vi "monitor_voltage.vi"() -> ()   [LabVIEW 2017]
uses:
  <vilib>/Instr/_visa.llb/VISA Configure Serial Port (Instr).vi
panel:
  in  "温度点维持时间（s）":dbl=30.0
  out "结束":bool
  in  "温度点（℃）":dbl[](array[numeric])=[70.0, 20.0, -40.0, -55.0, -40.0, 20.0, 70.0]
  in  "HP34401":refnum<visa-resource-name>
  out "XY图":cluster{dbl[], dbl[]}(graph)
  out "存储路径":string
  out "显示数据":i32(listbox)
  out "数据":string[][](array[string])
  in  "温度校验次数":dbl
  in  "实时温度(℃)":dbl
  in  "最低温度(℃)":dbl=-60.0
  in  "最高温度(℃)":dbl=75.0
  out "GWS":bool
  in  "GWS":refnum<visa-resource-name>
  in  "设定温度 (℃)":dbl
  in  "取点间隔 (S)":dbl
  in  "停止":bool
  in  "开始":bool
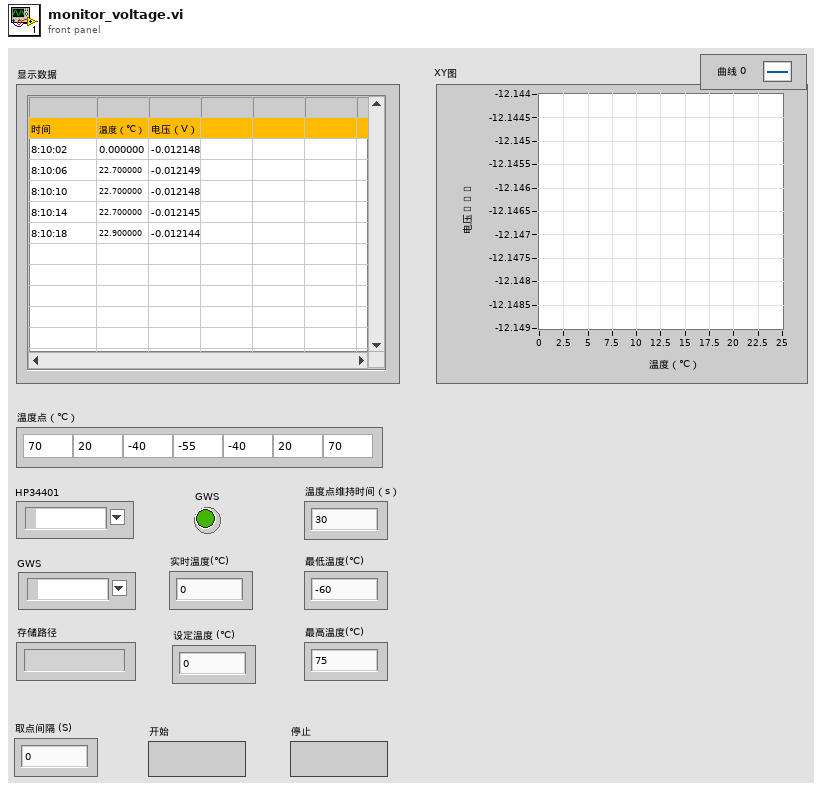
[diagram p1: front panel]
types:
  T1 = enum16{"open", "open or create", "create or replace", "create", "open (read-only)"}
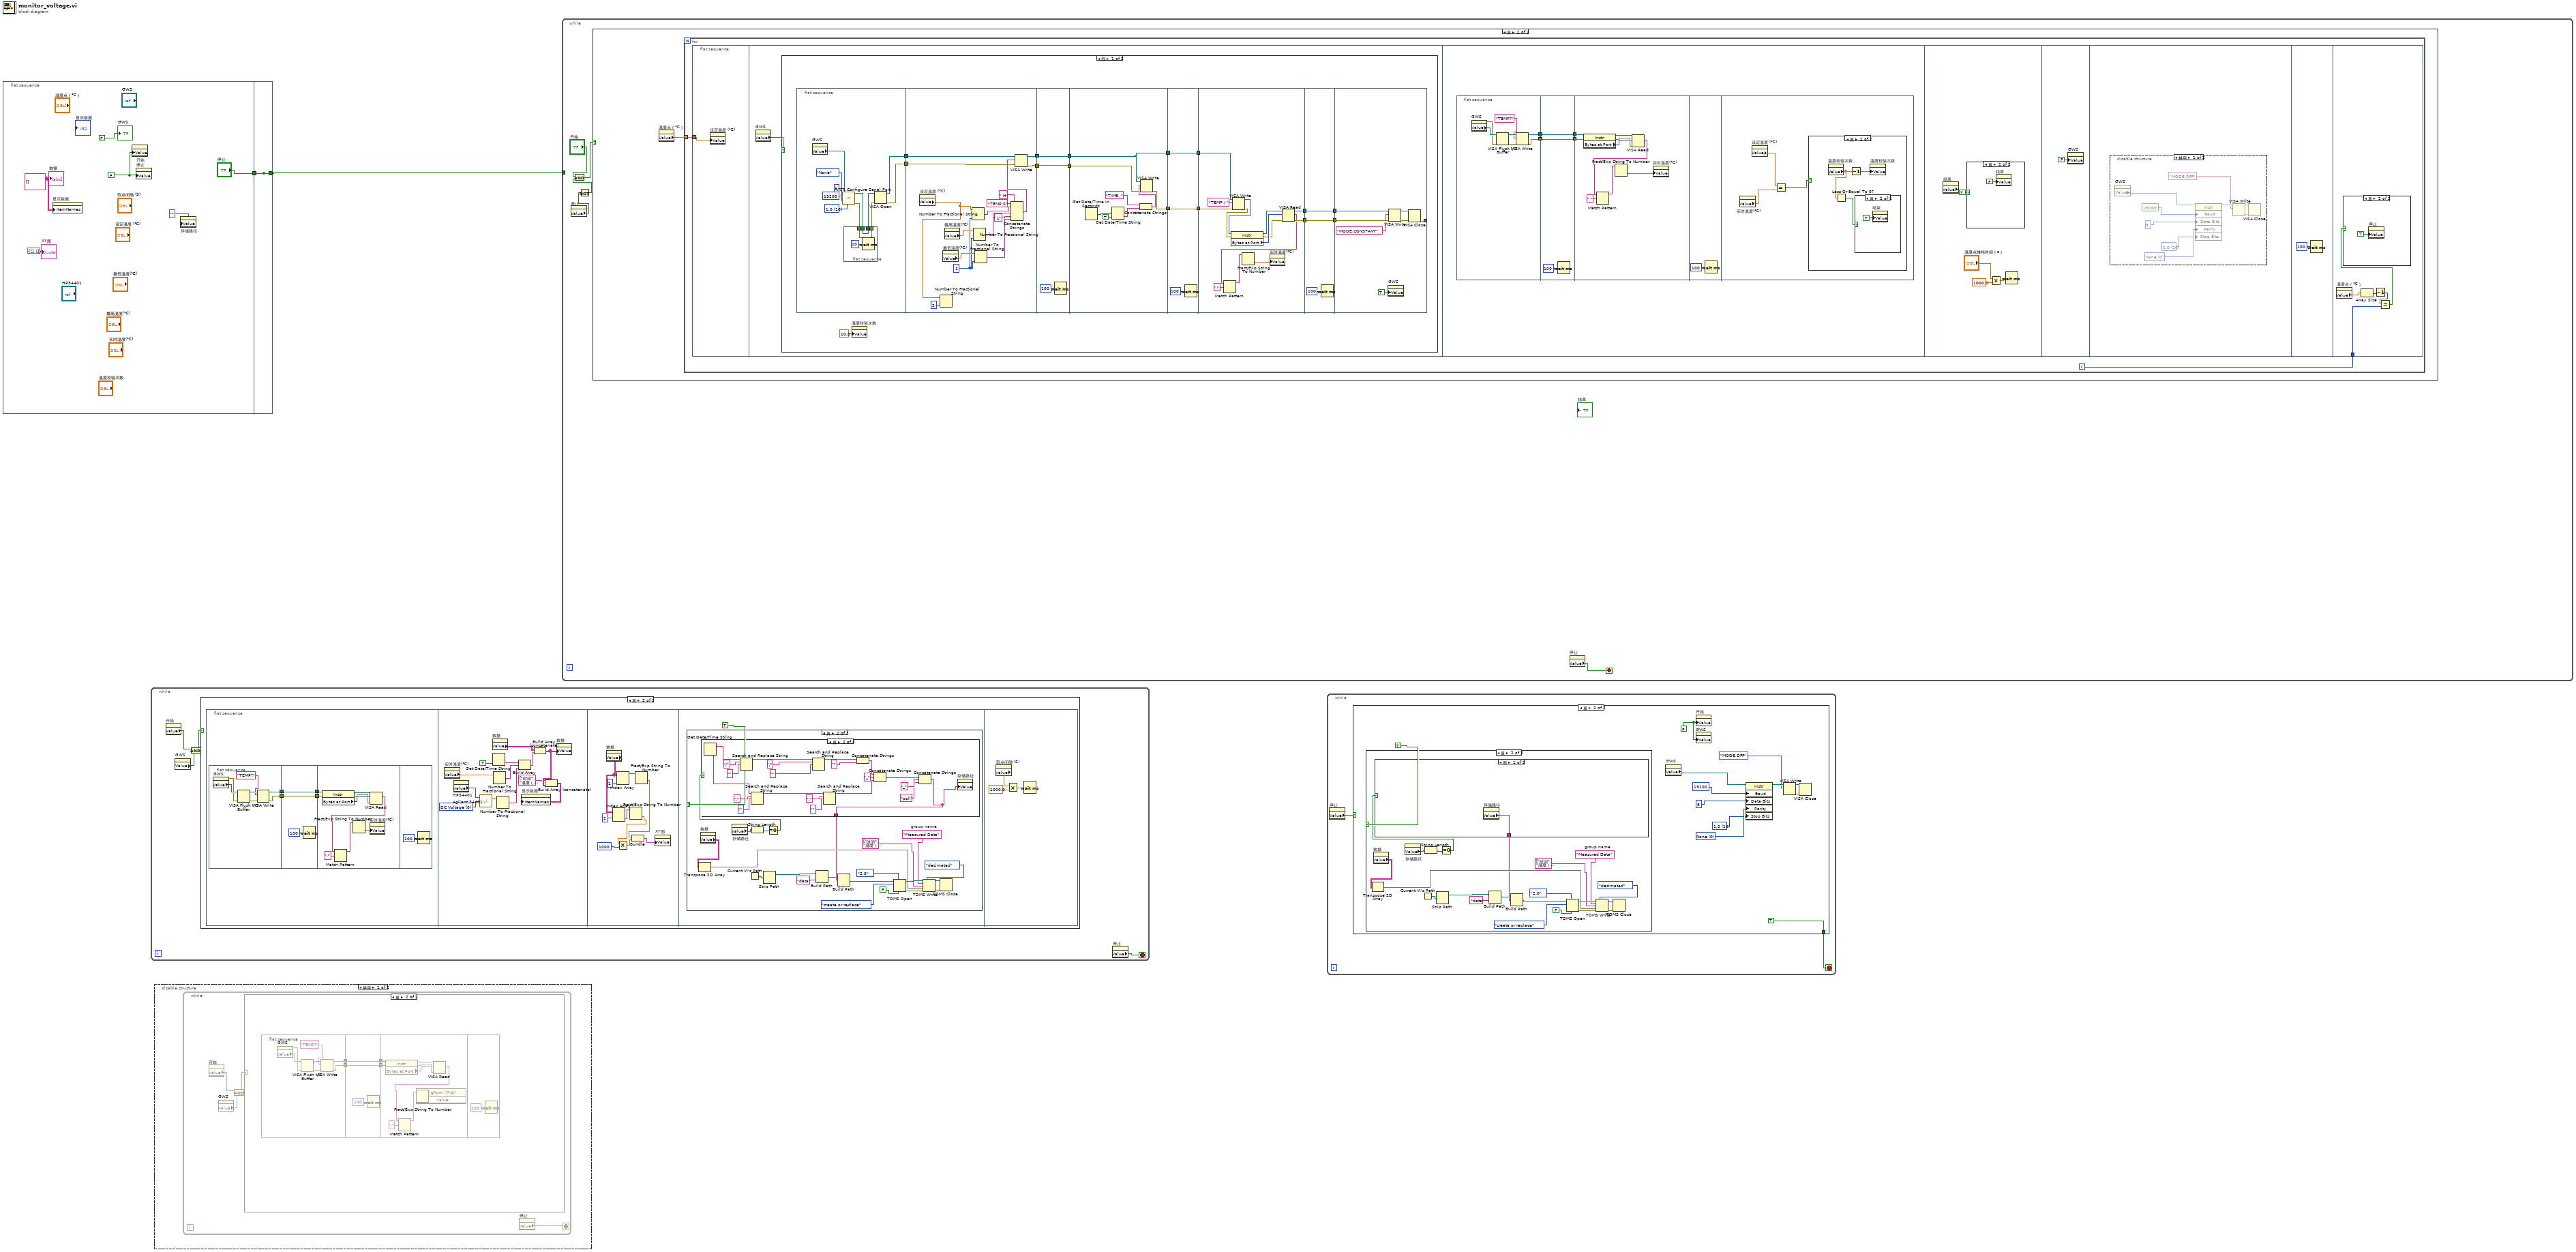
[diagram p0: block diagram]
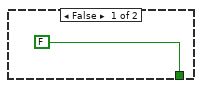
[diagram p4: hidden frame]
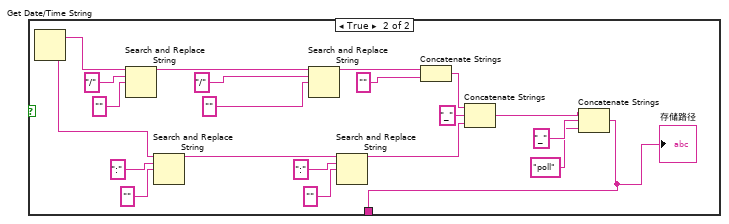
[diagram p6: hidden frame]
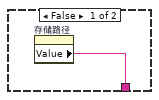
[diagram p9: hidden frame]
diagram:
  n1 = flat-sequence {
    tunnel: ["停止"] -> w2
    tunnel: [w9] -> _
    tunnel: w2 -> [w9]
    tunnel: [w9] -> w1
    frame #0 {
      w5 = FALSE ("停止")
      w8 = string[][] [] ("数据")
      n2 = property on="显示数据" class="MCListbox (严格)"("ItemNames"=w8) -> ()  [unwired: 2 in, 2 out]
      n3 = property on="开始" class="Bool (严格)"("Value"=w5) -> ()  [unwired: 2 in, 2 out]
      n4 = property on="停止" class="Bool (严格)"("Value"=w5) -> ()  [unwired: 2 in, 2 out]
      n5 = property on="存储路径" class="Str"("Value"="" ("存储路径")) -> ()  [unwired: 2 in, 2 out]
      "GWS" <- FALSE ("GWS")
      "数据" <- w8
      "XY图" <- cluster{dbl[], dbl[]} {[], []}
    }
    frame #1 {
    }
  }
  n6 = while {
    stop <- w10 stop-if-true
    n7 = property on="开始" class="Bool (严格)"() -> ("Value"=w11:bool)  [unwired: 2 in, 2 out]
    n8 = property on="GWS" class="Bool (严格)"() -> ("Value"=w13:bool)  [unwired: 2 in, 2 out]
    n9 = And(x=w11, y=w13) -> (x .and. y?=w12:bool)
    n10 = case shown="真" w12 {
      frame False {
      }
      frame True {
        n11 = flat-sequence {
          frame #0 {
            n12 = flat-sequence {
              tunnel: [w19] -> w17
              tunnel: [w18] -> w16
              tunnel: [w26] -> w15
              tunnel: w17 -> [w26]
              tunnel: [w25] -> w14
              tunnel: w16 -> [w25]
              tunnel: w15 -> [w36]
              tunnel: w14 -> [w35]
              frame #0 {
                n13 = property on="GWS" class="VISAName"() -> (error out=w23:errorcluster, "Value"=w24:refnum<visa-resource-name>)  [unwired: 2 in, 1 out]
                n14 = VISA Flush I/O Buffer(VISA resource name=w24, error in (no error)=w23) -> (VISA resource name out=w21:refnum<visa-resource-name>, error out=w22:errorcluster)  [unwired: 1 in]
                n15 = VISA Write(VISA resource name=w21, write buffer="TEMP?" ("写入缓冲区"), error in (no error)=w22) -> (VISA resource name out=w19:refnum<visa-resource-name>, error out=w18:errorcluster)  [unwired: 1 out]
              }
              frame #1 {
                n16 = Wait (ms)(milliseconds to wait=u32 100 ("等待时间（毫秒）")) -> ()  [unwired: 1 out]
              }
              frame #2 {
                n17 = property class="Instr"(reference=w36, error in=w35) -> (reference out=w34:refnum<visa-resource-name>, error out=w32:errorcluster, "Bytes at Port"=w33:u32)
                n18 = VISA Read(VISA resource name=w34, byte count=w33, error in (no error)=w32) -> (read buffer=w29:string)  [unwired: 3 out]
                n19 = Match Pattern(string=w29, regular expression="," ("正则表达式")) -> (before substring=w28:string)  [unwired: 1 in, 3 out]
                n20 = Fract/Exp String To Number(string=w28) -> (number=w31:dbl)  [unwired: 3 in, 1 out]
                n21 = property on="实时温度(℃)" class="DigNum (严格)"("Value"=w31) -> ()  [unwired: 2 in, 2 out]
              }
              frame #3 {
                n22 = Wait (ms)(milliseconds to wait=u32 100 ("等待时间（毫秒）")) -> ()  [unwired: 1 out]
              }
            }
          }
          frame #1 {
            w40 = u16 0 items=["DC Voltage", "AC Voltage", "2 - Wire Resistance", "4 - Wire Resistance", "DC Current", "AC Current", "Frequency", "Period", "Continuity", "Diode Checking", "VDC:VDC Ratio", "Temperature", "Capacitance"] ("Function (0: DC Voltage)")
            n23 = property on="实时温度(℃)" class="DigNum (严格)"() -> ("Value"=w49:dbl)  [unwired: 2 in, 2 out]
            n24 = property on="HP34401" class="VISAName"() -> ("Value"=w38:refnum<visa-resource-name>)  [unwired: 2 in, 2 out]
            n25 = call "Agilent 34401.vi"("Function (0: DC Voltage)"=w40, "VISA resource name"=w38) -> ("Measurement"=w50:dbl)  [unwired: 1 in, 1 out]
            n26 = property on="数据" class="Arr (严格)"() -> ("Value"=w44:string[][])  [unwired: 2 in, 2 out]
            n27 = Get Date/Time String(want seconds? (F)=TRUE ("disable buffering (T)")) -> (time string=w48:string)  [unwired: 2 in, 1 out]
            n28 = Number To Fractional String(number=w49) -> (F-format string=w47:string)  [unwired: 3 in]
            n29 = Number To Fractional String(number=w50) -> (F-format string=w46:string)  [unwired: 3 in]
            n30 = Build Array(w48, w47, w46) -> (w45:string[])
            n31 = Build Array (concatenate)(w44, w45) -> (w43:string[][])
            n32 = Build Array (concatenate)(string[] ["时间", "温度（℃）", "电压（V）"], w43) -> (w42:string[][])
            n33 = property on="显示数据" class="MCListbox (严格)"("ItemNames"=w42) -> ()  [unwired: 2 in, 2 out]
            n34 = property on="数据" class="Arr (严格)"("Value"=w43) -> ()  [unwired: 2 in, 2 out]
          }
          frame #2 {
            n35 = property on="数据" class="Arr (严格)"() -> ("Value"=w59:string[][])  [unwired: 2 in, 2 out]
            n36 = Index Array(array=w59, index (col)=2 ("禁用的索引 (列)")) -> (element=w55:string[])  [unwired: 1 in]
            n37 = Index Array(array=w59, index (col)=1 ("禁用的索引 (列)")) -> (element=w57:string[])  [unwired: 1 in]
            n38 = Fract/Exp String To Number(string=w55) -> (number=w52:dbl[])  [unwired: 3 in, 1 out]
            n39 = Multiply(x=w52, y=1000) -> (x*y=w53:dbl[])
            n40 = Fract/Exp String To Number(string=w57) -> (number=w56:dbl[])  [unwired: 3 in, 1 out]
            n41 = Bundle(w56, w53) -> (w54:cluster{dbl[], dbl[]})  [unwired: 1 in]
            n42 = property on="XY图" class="XYGraph (严格)"("Value"=w54) -> ()  [unwired: 2 in, 2 out]
          }
          frame #3 {
            n43 = case shown="真" TRUE {
              frame False {
              }
              frame True {
                w66 = "Measured Data"  # group name
                n44 = property on="数据" class="Arr (严格)"() -> ("Value"=w68:string[][])  [unwired: 2 in, 2 out]
                n45 = Transpose 2D Array(2D array=w68) -> (transposed array=w75:string[][])
                n46 = property on="存储路径" class="Str"() -> ("Value"=w65:string)  [unwired: 2 in, 2 out]
                n47 = Current VI's Path() -> (path=w69:path)
                n48 = String Length(string=w65) -> (length=w64:i32)
                n49 = Strip Path(path=w69) -> (stripped path=w79:path)  [unwired: 1 out]
                n50 = Equal To 0?(x=w64) -> (x = 0?=w63:bool)
                n51 = case shown="真" w63 {
                  tunnel: [w83 w84] -> w62
                  frame False {
                    n52 = property on="存储路径" class="Str"() -> ("Value"=w83:string)  [unwired: 2 in, 2 out]
                  }
                  frame True {
                    n53 = Get Date/Time String() -> (date string=w96:string, time string=w89:string)  [unwired: 3 in]
                    n54 = Search and Replace String(input string=w96, search string="/" ("搜索字符串"), replace string="" ("替换字符串(\"\")")) -> (result string=w102:string)  [unwired: 5 in, 3 out]
                    n55 = Search and Replace String(input string=w89, search string=":" ("搜索字符串"), replace string="" ("替换字符串(\"\")")) -> (result string=w93:string)  [unwired: 5 in, 3 out]
                    n56 = Search and Replace String(input string=w102, search string="/" ("搜索字符串"), replace string="" ("替换字符串(\"\")")) -> (result string=w99:string)  [unwired: 5 in, 3 out]
                    n57 = Search and Replace String(input string=w93, search string=":" ("搜索字符串"), replace string="" ("替换字符串(\"\")")) -> (result string=w88:string)  [unwired: 5 in, 3 out]
                    n58 = Concatenate Strings(w99, "" ("字符串")) -> (w97:string)
                    n59 = Concatenate Strings(w97, "_" ("字符串"), w88) -> (w86:string)
                    n60 = Concatenate Strings(w86, "_" ("字符串"), "poll" ("字符串")) -> (w84:string)
                    n61 = property on="存储路径" class="Str"("Value"=w84) -> ()  [unwired: 2 in, 2 out]
                  }
                }
                n62 = Build Path(base path=w79, name or relative path="data" ("字符串")) -> (appended path=w78:path)
                n63 = Build Path(base path=w78, name or relative path=w62) -> (appended path=w82:path)
                n64 = TDMS Open(6:FALSE ("disable buffering (T)"), 7:enum16{"1.0", "2.0"}."2.0" ("file format version (2.0)"), 10:T1."create or replace" ("operation"), 11:w82) -> (0:w80:errorcluster, 3:w77:refnum<k34>)  [unwired: 3 in]
                n65 = TDMS Write(0:w77, 1:enum16{"decimated", "interleaved"}."decimated" ("数据布局（0:降采样）"), 5:w66, 7:string[] ["时间", "温度（℃）", "电压（V）"], 9:w75, 11:w80) -> (4:w76:refnum<k34>, 15:w81:errorcluster)  [unwired: 2 out]
                n66 = TDMS Close(8:w81, 11:w76) -> ()  [unwired: 2 out]
              }
            }
          }
          frame #4 {
            n67 = property on="取点间隔 (S)" class="DigNum (严格)"() -> ("Value"=w107:dbl)  [unwired: 2 in, 2 out]
            n68 = Multiply(x=w107, y=1000.0) -> (x*y=w105:dbl)
            n69 = Wait (ms)(milliseconds to wait=w105) -> ()  [unwired: 1 out]
          }
        }
      }
    }
    n70 = property on="停止" class="Bool (严格)"() -> ("Value"=w10:bool)  [unwired: 2 in, 2 out]
  }
  n71 = disable-structure shown="禁用" {
    frame Disabled {
      n72 = while {
        stop <- w108 stop-if-true
        n73 = property on="开始" class="Bool (严格)"() -> ("Value"=w109:bool)  [unwired: 2 in, 2 out]
        n74 = property on="GWS" class="Bool (严格)"() -> ("Value"=w111:bool)  [unwired: 2 in, 2 out]
        n75 = And(x=w109, y=w111) -> (x .and. y?=w110:bool)
        n76 = case shown="真" w110 {
          frame False {
          }
          frame True {
            n77 = flat-sequence {
              tunnel: [w117] -> w115
              tunnel: [w116] -> w114
              tunnel: [w124] -> w113
              tunnel: w115 -> [w124]
              tunnel: [w123] -> w112
              tunnel: w114 -> [w123]
              tunnel: w113 -> [w134]
              tunnel: w112 -> [w133]
              frame #0 {
                n78 = property on="GWS" class="VISAName"() -> (error out=w121:errorcluster, "Value"=w122:refnum<visa-resource-name>)  [unwired: 2 in, 1 out]
                n79 = VISA Flush I/O Buffer(VISA resource name=w122, error in (no error)=w121) -> (VISA resource name out=w119:refnum<visa-resource-name>, error out=w120:errorcluster)  [unwired: 1 in]
                n80 = VISA Write(VISA resource name=w119, write buffer="TEMP?" ("写入缓冲区"), error in (no error)=w120) -> (VISA resource name out=w117:refnum<visa-resource-name>, error out=w116:errorcluster)  [unwired: 1 out]
              }
              frame #1 {
                n81 = Wait (ms)(milliseconds to wait=u32 100 ("等待时间（毫秒）")) -> ()  [unwired: 1 out]
              }
              frame #2 {
                n82 = property class="Instr"(reference=w134, error in=w133) -> (reference out=w132:refnum<visa-resource-name>, error out=w130:errorcluster, "Bytes at Port"=w131:u32)
                n83 = VISA Read(VISA resource name=w132, byte count=w131, error in (no error)=w130) -> (read buffer=w127:string)  [unwired: 3 out]
                n84 = Match Pattern(string=w127, regular expression="," ("正则表达式")) -> (before substring=w126:string)  [unwired: 1 in, 3 out]
                n85 = Fract/Exp String To Number(string=w126) -> (number=w129:dbl)  [unwired: 3 in, 1 out]
                n86 = property on="属性节点" class="DigNum (严格)"("Value"=w129) -> ()  [unwired: 2 in, 2 out]
              }
              frame #3 {
                n87 = Wait (ms)(milliseconds to wait=u32 100 ("等待时间（毫秒）")) -> ()  [unwired: 1 out]
              }
            }
          }
        }
        n88 = property on="停止" class="Bool (严格)"() -> ("Value"=w108:bool)  [unwired: 2 in, 2 out]
      }
    }
    frame Enabled {
    }
  }
  n89 = while {
    tunnel: w1 -> [_]
    stop <- w136 stop-if-true
    n90 = property on="停止" class="Bool (严格)"() -> ("Value"=w138:bool)  [unwired: 2 in, 2 out]
    n91 = Not(x=w138) -> (.not. x?=w137:bool)
    n92 = And(x="开始", y=w137) -> (x .and. y?=w139:bool)
    n93 = case shown="真" w139 {
      frame False {
      }
      frame True {
        n94 = property on="温度点（℃）" class="Arr (严格)"() -> ("Value"=w141:dbl[])  [unwired: 2 in, 2 out]
        n95 = for {
          tunnel: w141 -> [w142] mode=indexing
          i -> [w143]
          n96 = flat-sequence {
            tunnel: w142 -> [w144]
            tunnel: w143 -> [w277]
            frame #0 {
              n97 = property on="设定温度 (℃)" class="DigNum (严格)"("Value"=w144) -> ()  [unwired: 2 in, 2 out]
            }
            frame #1 {
              n98 = property on="GWS" class="Bool (严格)"() -> ("Value"=w145:bool)  [unwired: 2 in, 2 out]
              n99 = case shown="假" w145 {
                frame False {
                  n100 = flat-sequence {
                    tunnel: [w164] -> w160
                    tunnel: [w163] -> w159
                    tunnel: [w181] -> w158
                    tunnel: [w180] -> w157
                    tunnel: w160 -> [w178]
                    tunnel: w159 -> [w177]
                    tunnel: [w193] -> w156
                    tunnel: w158 -> [w193]
                    tunnel: [w192] -> w155
                    tunnel: w157 -> [w192]
                    tunnel: w156 -> [w195]
                    tunnel: w155 -> [w196]
                    tunnel: [w195] -> w154
                    tunnel: [w194] -> w153
                    tunnel: w154 -> [w203]
                    tunnel: [w203] -> w152
                    tunnel: [w202] -> w151
                    tunnel: w153 -> [w202]
                    tunnel: w152 -> [w216]
                    tunnel: w151 -> [w215]
                    tunnel: [w211] -> w150
                    tunnel: [w210] -> w149
                    tunnel: [w220] -> w148
                    tunnel: w150 -> [w220]
                    tunnel: w149 -> [w219]
                    tunnel: [w219] -> w147
                    tunnel: w148 -> [w227]
                    tunnel: w147 -> [w226]
                    tunnel: [w222] -> _
                    frame #0 {
                      w168 = u16 10 items=["1.0"=10, "1.5"=15, "2.0"=20] ("stop bits (10: 1 bit)")
                      n101 = property on="GWS" class="VISAName"() -> ("Value"=w167:refnum<visa-resource-name>)  [unwired: 2 in, 2 out]
                      n102 = call-poly "VISA Configure Serial Port"("VISA resource name"=w167, "baud rate (9600)"=u32 19200, "data bits (8)"=u16 8, "parity (0:none)"=enum16{"None", "Odd", "Even", "Mark", "Space"}."None", "stop bits (10: 1 bit)"=w168) -> ("VISA resource name out"=w162:refnum<visa-resource-name>, "error out"=w166:errorcluster)  [unwired: 9 in]
                      n103 = flat-sequence {
                        tunnel: w166 -> [w173]
                        tunnel: [w173] -> w165
                        tunnel: w162 -> [w172]
                        tunnel: [w172] -> w161
                        frame #0 {
                          n104 = Wait (ms)(milliseconds to wait=u32 20 ("等待时间（毫秒）")) -> ()  [unwired: 1 out]
                        }
                      }
                      n105 = VISA Open(error in (no error)=w165, VISA resource name=w161) -> (VISA resource name=w164:refnum<visa-resource-name>, error out=w163:errorcluster)  [unwired: 3 in]
                    }
                    frame #1 {
                      w185 = i16 1 ("精度(6)")
                      n106 = property on="设定温度 (℃)" class="DigNum (严格)"() -> ("Value"=w175:dbl)  [unwired: 2 in, 2 out]
                      n107 = Number To Fractional String(number=w175, precision (6)=i16 2 ("精度(6)")) -> ()  [unwired: 2 in, 1 out]
                      n108 = property on="最低温度(℃)" class="DigNum (严格)"() -> ("Value"=w187:dbl)  [unwired: 2 in, 2 out]
                      n109 = property on="最高温度(℃)" class="DigNum (严格)"() -> ("Value"=w186:dbl)  [unwired: 2 in, 2 out]
                      n110 = Number To Fractional String(number=w175, precision (6)=w185) -> (F-format string=w190:string)  [unwired: 2 in]
                      n111 = Number To Fractional String(number=w186, precision (6)=w185) -> (F-format string=w188:string)  [unwired: 2 in]
                      n112 = Number To Fractional String(number=w187, precision (6)=w185) -> (F-format string=w189:string)  [unwired: 2 in]
                      n113 = Concatenate Strings("TEMP,S" ("字符串"), w190, " H" ("字符串"), w188, " L" ("字符串"), w189) -> (w179:string)
                      n114 = VISA Write(VISA resource name=w178, write buffer=w179, error in (no error)=w177) -> (VISA resource name out=w181:refnum<visa-resource-name>, error out=w180:errorcluster)  [unwired: 1 out]
                    }
                    frame #2 {
                      n115 = Wait (ms)(milliseconds to wait=u32 100 ("等待时间（毫秒）")) -> ()  [unwired: 1 out]
                    }
                    frame #3 {
                      n116 = Get Date/Time In Seconds() -> (seconds since 1Jan1904=w199:timestamp)
                      n117 = Get Date/Time String(seconds (now)=w199, want seconds? (F)=TRUE ("需要秒？(F)")) -> (time string=w201:string)  [unwired: 1 in, 1 out]
                      n118 = Concatenate Strings("TIME, " ("字符串"), w201) -> (w197:string)
                      n119 = VISA Write(VISA resource name=w195, write buffer=w197, error in (no error)=w196) -> (error out=w194:errorcluster)  [unwired: 2 out]
                    }
                    frame #4 {
                      n120 = Wait (ms)(milliseconds to wait=u32 100 ("等待时间（毫秒）")) -> ()  [unwired: 1 out]
                    }
                    frame #5 {
                      n121 = VISA Write(VISA resource name=w216, write buffer="TEMP？" ("写入缓冲区"), error in (no error)=w215) -> (VISA resource name out=w217:refnum<visa-resource-name>, error out=w212:errorcluster)  [unwired: 1 out]
                      n122 = property class="Instr"(reference=w217, error in=w212) -> (reference out=w214:refnum<visa-resource-name>, error out=w209:errorcluster, "Bytes at Port"=w213:u32)
                      n123 = VISA Read(VISA resource name=w214, byte count=w213, error in (no error)=w209) -> (VISA resource name out=w211:refnum<visa-resource-name>, read buffer=w205:string, error out=w210:errorcluster)  [unwired: 1 out]
                      n124 = Match Pattern(string=w205, regular expression="," ("正则表达式")) -> (before substring=w206:string)  [unwired: 1 in, 3 out]
                      n125 = Fract/Exp String To Number(string=w206) -> (number=w208:dbl)  [unwired: 3 in, 1 out]
                      n126 = property on="实时温度(℃)" class="DigNum (严格)"("Value"=w208) -> ()  [unwired: 2 in, 2 out]
                    }
                    frame #6 {
                      n127 = Wait (ms)(milliseconds to wait=u32 100 ("等待时间（毫秒）")) -> ()  [unwired: 1 out]
                    }
                    frame #7 {
                      n128 = property on="GWS" class="Bool (严格)"("Value"=TRUE ("GWS")) -> ()  [unwired: 2 in, 2 out]
                      n129 = VISA Write(VISA resource name=w227, write buffer="MODE,CONSTANT" ("写入缓冲区"), error in (no error)=w226) -> (VISA resource name out=w224:refnum<visa-resource-name>, error out=w223:errorcluster)  [unwired: 1 out]
                      n130 = VISA Close(VISA resource name=w224, error in (no error)=w223) -> (error out=w222:errorcluster)
                    }
                  }
                  n131 = property on="温度校验次数" class="DigNum (严格)"("Value"=10.0 ("温度校验次数")) -> ()  [unwired: 2 in, 2 out]
                }
                frame True {
                }
              }
            }
            frame #2 {
              n132 = flat-sequence {
                tunnel: [w234] -> w232
                tunnel: [w233] -> w231
                tunnel: [w241] -> w230
                tunnel: w232 -> [w241]
                tunnel: [w240] -> w229
                tunnel: w231 -> [w240]
                tunnel: w230 -> [w251]
                tunnel: w229 -> [w250]
                frame #0 {
                  n133 = property on="GWS" class="VISAName"() -> (error out=w238:errorcluster, "Value"=w239:refnum<visa-resource-name>)  [unwired: 2 in, 1 out]
                  n134 = VISA Flush I/O Buffer(VISA resource name=w239, error in (no error)=w238) -> (VISA resource name out=w236:refnum<visa-resource-name>, error out=w237:errorcluster)  [unwired: 1 in]
                  n135 = VISA Write(VISA resource name=w236, write buffer="TEMP?" ("写入缓冲区"), error in (no error)=w237) -> (VISA resource name out=w234:refnum<visa-resource-name>, error out=w233:errorcluster)  [unwired: 1 out]
                }
                frame #1 {
                  n136 = Wait (ms)(milliseconds to wait=u32 100 ("等待时间（毫秒）")) -> ()  [unwired: 1 out]
                }
                frame #2 {
                  n137 = property class="Instr"(reference=w251, error in=w250) -> (reference out=w249:refnum<visa-resource-name>, error out=w247:errorcluster, "Bytes at Port"=w248:u32)
                  n138 = VISA Read(VISA resource name=w249, byte count=w248, error in (no error)=w247) -> (read buffer=w244:string)  [unwired: 3 out]
                  n139 = Match Pattern(string=w244, regular expression="," ("正则表达式")) -> (before substring=w243:string)  [unwired: 1 in, 3 out]
                  n140 = Fract/Exp String To Number(string=w243) -> (number=w246:dbl)  [unwired: 3 in, 1 out]
                  n141 = property on="实时温度(℃)" class="DigNum (严格)"("Value"=w246) -> ()  [unwired: 2 in, 2 out]
                }
                frame #3 {
                  n142 = Wait (ms)(milliseconds to wait=u32 100 ("等待时间（毫秒）")) -> ()  [unwired: 1 out]
                }
                frame #4 {
                  n143 = property on="实时温度(℃)" class="DigNum (严格)"() -> ("Value"=w255:dbl)  [unwired: 2 in, 2 out]
                  n144 = property on="设定温度 (℃)" class="DigNum (严格)"() -> ("Value"=w254:dbl)  [unwired: 2 in, 2 out]
                  n145 = Equal?(x=w254, y=w255) -> (x = y?=w253:bool)
                  n146 = case shown="真" w253 {
                    frame False {
                    }
                    frame True {
                      n147 = property on="温度校验次数" class="DigNum (严格)"() -> ("Value"=w256:dbl)  [unwired: 2 in, 2 out]
                      n148 = Less Or Equal To 0?(x=w256) -> (x <= 0?=w257:bool)
                      n149 = Decrement(x=w256) -> (x-1=w258:dbl)
                      n150 = case shown="真" w257 {
                        frame False {
                        }
                        frame True {
                          n151 = property on="结束" class="Bool (严格)"("Value"=TRUE ("结束")) -> ()  [unwired: 2 in, 2 out]
                        }
                      }
                      n152 = property on="温度校验次数" class="DigNum (严格)"("Value"=w258) -> ()  [unwired: 2 in, 2 out]
                    }
                  }
                }
              }
            }
            frame #3 {
              n153 = property on="结束" class="Bool (严格)" props=["Value"]() -> ()  [unwired: 2 in, 3 out]
              n154 = case shown="真" TRUE {
                frame False {
                }
                frame True {
                  n155 = property on="结束" class="Bool (严格)"("Value"=FALSE ("结束")) -> ()  [unwired: 2 in, 2 out]
                }
              }
              n156 = Multiply(x="温度点维持时间（s）", y=1000.0) -> (x*y=w261:dbl)
              n157 = Wait (ms)(milliseconds to wait=w261) -> ()  [unwired: 1 out]
            }
            frame #4 {
              n158 = property on="GWS" class="Bool (严格)"("Value"=FALSE ("结束")) -> ()  [unwired: 2 in, 2 out]
            }
            frame #5 {
              n159 = disable-structure shown="禁用" {
                frame Disabled {
                  w266 = u16 10 items=["1.0"=10, "1.5"=15, "2.0"=20] ("Serial Settings:Stop Bits")
                  w267 = u16 0 items=["None", "Odd", "Even", "Mark", "Space"] ("Serial Settings:Parity")
                  n160 = property on="GWS" class="VISAName"() -> ("Value"=w274:refnum<visa-resource-name>)  [unwired: 2 in, 2 out]
                  n161 = property class="Instr"(reference=w274, "Baud"=u32 19200 ("Serial Settings:Baud Rate"), "Data Bits"=u16 8 ("Serial Settings:Data Bits"), "Parity"=w267, "Stop Bits"=w266) -> (reference out=w271:refnum<visa-resource-name>)  [unwired: 1 in, 1 out]
                  n162 = VISA Write(VISA resource name=w271, write buffer="MODE,OFF" ("写入缓冲区")) -> (VISA resource name out=w273:refnum<visa-resource-name>, error out=w272:errorcluster)  [unwired: 1 in, 1 out]
                  n163 = VISA Close(VISA resource name=w273, error in (no error)=w272) -> ()  [unwired: 1 out]
                }
                frame Enabled {
                }
              }
            }
            frame #6 {
              n164 = Wait (ms)(milliseconds to wait=u32 100 ("等待时间（毫秒）")) -> ()  [unwired: 1 out]
            }
            frame #7 {
              n165 = property on="温度点（℃）" class="Arr (严格)"() -> ("Value"=w280:dbl[])  [unwired: 2 in, 2 out]
              n166 = Array Size(array=w280) -> (size(s)=w279:i32)
              n167 = Decrement(x=w279) -> (x-1=w278:i32)
              n168 = Equal?(x=w278, y=w277) -> (x = y?=w276:bool)
              n169 = case shown="真" w276 {
                frame False {
                }
                frame True {
                  n170 = property on="停止" class="Bool (严格)"("Value"=TRUE ("恒温开始")) -> ()  [unwired: 2 in, 2 out]
                }
              }
            }
          }
        }
      }
    }
    n171 = property on="停止" class="Bool (严格)"() -> ("Value"=w136:bool)  [unwired: 2 in, 2 out]
  }
  n172 = while {
    stop <- w282 stop-if-true
    n173 = property on="停止" class="Bool (严格)"() -> ("Value"=w283:bool)  [unwired: 2 in, 2 out]
    n174 = case shown="真" w283 {
      tunnel: [FALSE TRUE] -> w282
      frame False {
      }
      frame True {
        w287 = FALSE ("开始")
        w288 = u16 10 items=["1.0"=10, "1.5"=15, "2.0"=20] ("Serial Settings:Stop Bits")
        w289 = u16 0 items=["None", "Odd", "Even", "Mark", "Space"] ("Serial Settings:Parity")
        n175 = case shown="真" TRUE {
          frame False {
          }
          frame True {
            w301 = "Measured Data"  # group name
            n176 = property on="数据" class="Arr (严格)"() -> ("Value"=w303:string[][])  [unwired: 2 in, 2 out]
            n177 = Transpose 2D Array(2D array=w303) -> (transposed array=w310:string[][])
            n178 = property on="存储路径" class="Str"() -> ("Value"=w300:string)  [unwired: 2 in, 2 out]
            n179 = Current VI's Path() -> (path=w304:path)
            n180 = String Length(string=w300) -> (length=w299:i32)
            n181 = Strip Path(path=w304) -> (stripped path=w314:path)  [unwired: 1 out]
            n182 = Equal To 0?(x=w299) -> (x = 0?=w298:bool)
            n183 = case shown="假" w298 {
              tunnel: [w318 w319] -> w297
              frame False {
                n184 = property on="存储路径" class="Str"() -> ("Value"=w318:string)  [unwired: 2 in, 2 out]
              }
              frame True {
                n185 = Get Date/Time String() -> (date string=w331:string, time string=w324:string)  [unwired: 3 in]
                n186 = Search and Replace String(input string=w331, search string="/" ("搜索字符串"), replace string="" ("替换字符串(\"\")")) -> (result string=w337:string)  [unwired: 5 in, 3 out]
                n187 = Search and Replace String(input string=w324, search string=":" ("搜索字符串"), replace string="" ("替换字符串(\"\")")) -> (result string=w328:string)  [unwired: 5 in, 3 out]
                n188 = Search and Replace String(input string=w337, search string="/" ("搜索字符串"), replace string="" ("替换字符串(\"\")")) -> (result string=w334:string)  [unwired: 5 in, 3 out]
                n189 = Search and Replace String(input string=w328, search string=":" ("搜索字符串"), replace string="" ("替换字符串(\"\")")) -> (result string=w323:string)  [unwired: 5 in, 3 out]
                n190 = Concatenate Strings(w334, "" ("字符串")) -> (w332:string)
                n191 = Concatenate Strings(w332, "_" ("字符串"), w323) -> (w321:string)
                n192 = Concatenate Strings(w321, "_" ("字符串"), "poll" ("字符串")) -> (w319:string)
                "存储路径" <- w319
              }
            }
            n193 = Build Path(base path=w314, name or relative path="data" ("字符串")) -> (appended path=w313:path)
            n194 = Build Path(base path=w313, name or relative path=w297) -> (appended path=w317:path)
            n195 = TDMS Open(6:FALSE ("disable buffering (T)"), 7:enum16{"1.0", "2.0"}."2.0" ("file format version (2.0)"), 10:T1."create or replace" ("operation"), 11:w317) -> (0:w315:errorcluster, 3:w312:refnum<k34>)  [unwired: 3 in]
            n196 = TDMS Write(0:w312, 1:enum16{"decimated", "interleaved"}."decimated" ("数据布局（0:降采样）"), 5:w301, 7:string[] ["时间", "温度（℃）", "电压（V）"], 9:w310, 11:w315) -> (4:w311:refnum<k34>, 15:w316:errorcluster)  [unwired: 2 out]
            n197 = TDMS Close(8:w316, 11:w311) -> ()  [unwired: 2 out]
          }
        }
        n198 = property on="GWS" class="VISAName"() -> ("Value"=w296:refnum<visa-resource-name>)  [unwired: 2 in, 2 out]
        n199 = property on="开始" class="Bool (严格)"("Value"=w287) -> ()  [unwired: 2 in, 2 out]
        n200 = property on="GWS" class="Bool (严格)"("Value"=w287) -> ()  [unwired: 2 in, 2 out]
        n201 = property class="Instr"(reference=w296, "Baud"=u32 19200 ("Serial Settings:Baud Rate"), "Data Bits"=u16 8 ("Serial Settings:Data Bits"), "Parity"=w289, "Stop Bits"=w288) -> (reference out=w293:refnum<visa-resource-name>)  [unwired: 1 in, 1 out]
        n202 = VISA Write(VISA resource name=w293, write buffer="MODE,OFF" ("写入缓冲区")) -> (VISA resource name out=w295:refnum<visa-resource-name>, error out=w294:errorcluster)  [unwired: 1 in, 1 out]
        n203 = VISA Close(VISA resource name=w295, error in (no error)=w294) -> ()  [unwired: 1 out]
      }
    }
  }
